vi "StateScalarStateColorStateName.vi"() -> ()   [LabVIEW 2013, in "examples.lvlib"]
uses:
  examples.lvlib
  vis/lv-2013/tango_vi.llb/_TangoReadStateScalarAttribute.vi
  vis/lv-2013/tango_vi.llb/tango.lvlib
panel:
  in  "<TangoTest> device name":string="sys/tg_test/1"
  out "State Name":string
  out "State Color":u32(colorbox)=16448250
  out "State Code":u32
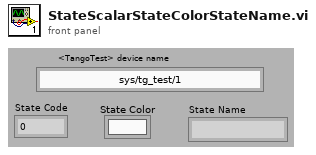
[diagram p1: front panel]
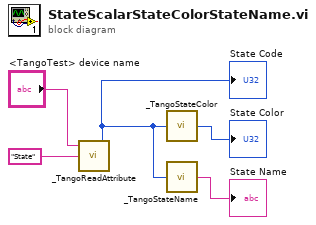
[diagram p0: block diagram]
diagram:
  n1 = call-poly "_TangoReadAttribute.vi"("attribute name"="State", "device name"="<TangoTest> device name") -> ("value"=w2:u32)  [unwired: 1 in, 2 out]
  "State Code" <- w2
  n2 = call "_TangoStateColor.vi"("State"=w2) -> ("State Color"=→"State Color":u32)
  n3 = call "_TangoStateName.vi"("State"=w2) -> ("State Name"=→"State Name":string)
